vi "setLUT_action.vi"(0 "HGF_ImaqFg in":refnum<class "HGF_ImaqFg.lvclass">, 1 "Tap 0 LUT (Red)":u16[](array[numeric]), 2 "Tap 1 LUT (Green)":u16[](array[numeric]), 3 "Tap 2 LUT (Blue)":u16[](array[numeric]), 4 "Tap 3 LUT":u16[](array[numeric]), 5 "error in (no error)":errorcluster) -> (14 "HGF_ImaqFg out":refnum<class "HGF_ImaqFg.lvclass">, 19 "error out":errorcluster)   [LabVIEW 2014, in "HGF_IMAQ.lvlib" / "HGF_ImaqFg.lvclass"]
doc: "Downloads a custom lookup table (LUT) to an image acquisition device. This VI can download 8-bit or 16-bit LUTs for analog or digital devices. If the image acquisition device has multiple LUTs, you can input all of the LUTs into this VI. Call this VI before starting the acquisition."
uses:
  HGF_ImaqFg.lvclass
  HGF_IMAQDevice/HGF_IMAQDevice.lvclass
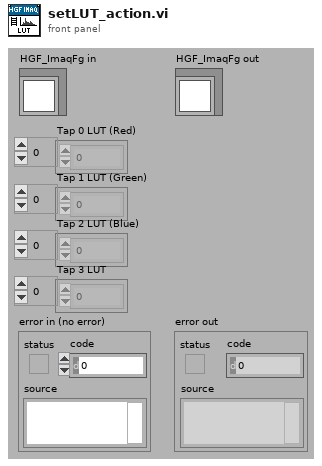
[diagram p1: front panel]
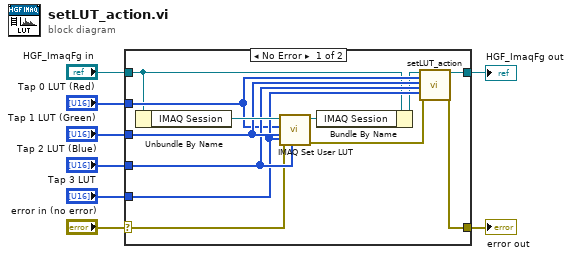
[diagram p0: block diagram]
diagram:
  n1 = case shown="No Error" "error in (no error)" {
    selector: "error in (no error)" -> [w14 w21]
    tunnel: "HGF_ImaqFg in" -> [w10 w22]
    tunnel: [w20 w22] -> w7
    tunnel: "Tap 0 LUT (Red)" -> [w15 _]
    tunnel: "Tap 1 LUT (Green)" -> [w18 _]
    tunnel: "Tap 2 LUT (Blue)" -> [w17 _]
    tunnel: "Tap 3 LUT" -> [w16 _]
    tunnel: [w12 w21] -> w2
    frame No Error {
      n2 = Unbundle By Name(w10) -> ("IMAQ Session"=w19:refnum<k11>)
      n3 = call <vilib>:"IMAQ Set User LUT.vi"("Tap 3 LUT"=w16, "Tap 2 LUT (Blue)"=w17, "error in (no error)"=w14, "Tap 1 LUT (Green)"=w18, "Tap 0 LUT (Red)"=w15, "IMAQ Session In"=w19) -> ("error out"=w13:errorcluster, "IMAQ Session Out"=w11:refnum<k11>)  [unwired: 4 in]
      n4 = Bundle By Name(cluster=w10, "IMAQ Session"=w11) -> (w9:refnum<class "HGF_ImaqFg.lvclass">)
      n5 = call-parent "setLUT_action.vi"("HGF_IMAQDevice in"=w9, "Tap 0 LUT (Red)"=w15, "Tap 1 LUT (Green)"=w18, "Tap 2 LUT (Blue)"=w17, "Tap 3 LUT"=w16, "error in (no error)"=w13) -> ("HGF_IMAQDevice out"=w20:refnum<class "HGF_ImaqFg.lvclass">, "error out"=w12:errorcluster)  [unwired: 12 in]
    }
    frame Error {
    }
  }
  "error out" <- w2
  "HGF_ImaqFg out" <- w7
